vi "LFU Create File Handle__ogtk.vi"(4 "error in (no error)":errorcluster, 6 "handle":u32, 7 "file path":path) -> (0 "error out":errorcluster, 3 "file refnum":refnum<file>)   [LabVIEW 2020]
doc: "Low level utility function tocreate a LabVIEW file handle from a platform API specific file handle."
panel:
  # "[OpenG VI Tags] ***Do Not Remove***"
  # "LFU Create File Handle.vi\n\nPlease visit http://www.OpenG.org to learn about the\nOpen Source LabVIEW software movement.\n\nNOTICE -- YOU MUST LEAVE THIS NOTICE IN PLACE.  PER THE TERMS OF THE LICENSE BELOW, YOU MAY SUBLICENSE THIS SOFTWARE \nIN ANY WAY THAT DOES NOT CONFLICT WITH THIS LICENSE.\n\n### BSD License (http://www.opensource.org/licenses/bsd-license.php) Begin ###\n\nCopyright (c) 2003, Rolf Kalbermatter <rolf.kalbermatter@citeng.com>\n\nAll rights reserved.\n\nRedistribution and use in source and binary forms, with or without modification, are permitted provided that the following conditions are met:\n\n    * Redistributions of source code must retain the above copyright notice, this list of conditions and the following disclaimer.\n    * Redistributions in binary form must reproduce the above copyright notice, this list of conditions and the following disclaimer in the \n       documentation and/or other materials provided with the distribution.\n    * Neither the name of SciWare, James Kring, Inc., nor the names of its contributors may be used to endorse or promote products derived \n       from this software without specific prior written permission.\n\nTHIS SOFTWARE IS PROVIDED BY THE COPYRIGHT HOLDERS AND CONTRIBUTORS \"AS IS\" AND ANY EXPRESS OR IMPLIED WARRANTIES, \nINCLUDING, BUT NOT LIMITED TO, THE IMPLIED WARRANTIES OF MERCHANTABILITY AND FITNESS FOR A PARTICULAR PURPOSE ARE \nDISCLAIMED. IN NO EVENT SHALL THE COPYRIGHT OWNER OR CONTRIBUTORS BE LIABLE FOR ANY DIRECT, INDIRECT, INCIDENTAL,\n SPECIAL, EXEMPLARY, OR CONSEQUENTIAL DAMAGES (INCLUDING, BUT NOT LIMITED TO, PROCUREMENT OF SUBSTITUTE GOODS OR \nSERVICES; LOSS OF USE, DATA, OR PROFITS; OR BUSINESS INTERRUPTION) HOWEVER CAUSED AND ON ANY THEORY OF LIABILITY, \nWHETHER IN CONTRACT, STRICT LIABILITY, OR TORT (INCLUDING NEGLIGENCE OR OTHERWISE) ARISING IN ANY WAY OUT OF THE USE \nOF THIS SOFTWARE, EVEN IF ADVISED OF THE POSSIBILITY OF SUCH DAMAGE.\n\n### BSD License End ###"
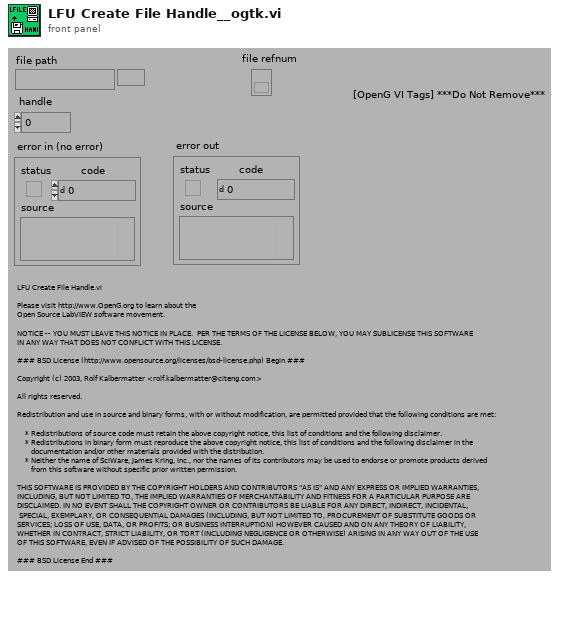
[diagram p1: front panel]
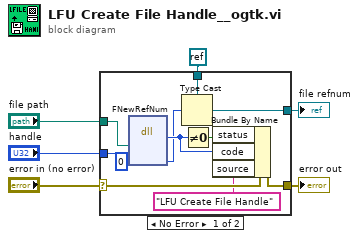
[diagram p0: block diagram]
diagram:
  n1 = case shown="No Error" "error in (no error)" {
    selector: "error in (no error)" -> [w17 w19]
    tunnel: "handle" -> [w10 _]
    tunnel: [w16 w19] -> w5
    tunnel: [w12 w18] -> w3
    tunnel: refnum<k0> refnum -> [w11 w18]
    tunnel: "file path" -> [w8 _]
    frame No Error {
      n2 = dll-call lib="LabVIEW" fn="FNewRefNum"("file path"=w8, "refNum"=w10, "fd"=u32 0) -> (w13:i32, "fd"=w7:u32)  [unwired: 5 in, 2 out]
      n3 = Type Cast(type=w11, x=w7) -> (*(type *) &x=w12:refnum<k0>)
      n4 = Not Equal To 0?(x=w13) -> (x != 0?=w14:bool)
      n5 = Bundle By Name(cluster=w17, "status"=w14, "code"=w13, "source"="LFU Create File Handle") -> (w16:errorcluster)
    }
    frame Error {
      (unwired) u32 0 ("fd")
    }
  }
  "file refnum" <- w3
  "error out" <- w5
